vi "CANTESTDouble.vi"(6 "Data Input(Hex)":string="000007d100000000", 8 "错误输入（无错误）":errorcluster, 9 "ID(Hex 高位有效)":string="00000182", 10 "CANChannel":u32) -> (0 "错误输出":errorcluster, 3 "帧数据":string)   [LabVIEW 2013]
uses:
  InitConfig.ctl
  DevType.ctl
panel:
  out "Result":bool
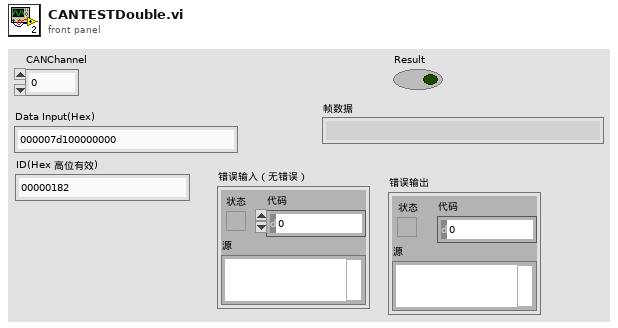
[diagram p1: front panel]
types:
  T1 = typedef "DevType.ctl" = u16
  T2 = typedef "InitConfig.ctl" = cluster{"AccCode":u32, "AccMask":u32, "Reserved":u32, "Filter":u8, "kCanBaud":u8, "Timing0":u8, "Timing1":u8, "Mode":u8, "CanRx_IER":u8}
  T3 = cluster{"ID":u8, u8, u8, u8, "TimeStamp":u32, "TimeFlag":u8, "SendType":u8, "RemoteFlag":u8, "ExternFlag":u8, "DataLen":u8, "Byte0":u8, "Byte1":u8, "Byte2":u8, "Byte3":u8, "Byte4":u8, "Byte5":u8, "Byte6":u8, "Byte7":u8, "Channel":u8, u8, u8}
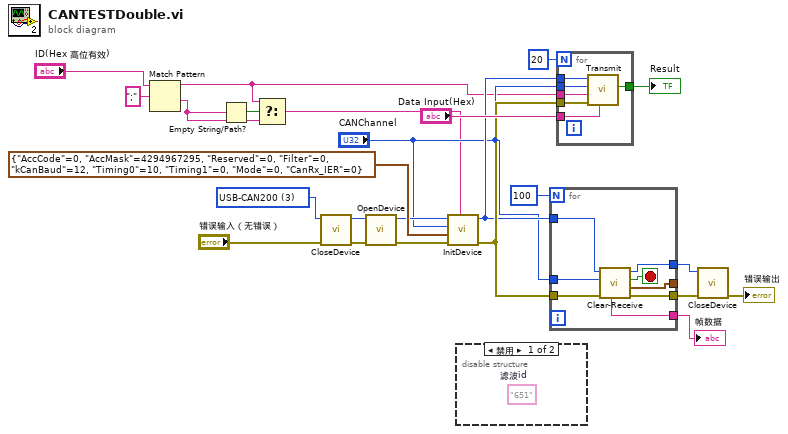
[diagram p0: block diagram]
diagram:
  w23 = T1 3 items=["PCI-CAN200"=7, "USB-CAN"=2, "USB-CAN200"=3] ("DeviceType")
  n1 = Match Pattern(string="ID(Hex 高位有效)", regular expression=";" ("正则表达式")) -> (before substring=w3:string, after substring=w2:string)  [unwired: 1 in, 2 out]
  n2 = Empty String/Path?(string/path=w2) -> (empty?=w4:bool)
  n3 = Select(t=w3, s=w4, f=w2) -> (s? t:f=w1:string)
  n4 = call "CloseDevice.vi"("错误输入（无错误）"="错误输入（无错误）", "DeviceType"=w23) -> ("错误输出"=w17:errorcluster, "DeviceTypeOut"=w22:u16)  [unwired: 7 in, 1 out]
  n5 = call "OpenDevice.vi"("错误输入（无错误）"=w17, "DeviceType"=w22) -> ("错误输出"=w18:errorcluster, "DeviceTypeOut"=w21:u16)  [unwired: 7 in, 1 out]
  n6 = call "InitDevice.vi"("ID(Hex 高位有效)"=w1, "错误输入（无错误）"=w18, "InitConfig"=T2 {"AccCode"=0, "AccMask"=4294967295, "Reserved"=0, "Filter"=0, "kCanBaud"=12, "Timing0"=10, "Timing1"=0, "Mode"=0, "CanRx_IER"=0}, "CanChannel"="CANChannel", "DeviceType"=w21) -> ("错误输出"=w12:errorcluster, "DeviceTypeOut"=w9:u16)  [unwired: 4 in, 1 out]
  n7 = disable-structure shown="禁用" {
    frame Disabled {
      (unwired) "651"  # 滤波id
    }
    frame Enabled {
    }
  }
  n8 = for {
    N: 100 -> [_]
    tunnel: "CANChannel" -> [w32]
    tunnel: w12 -> [w31]
    tunnel: [w29] -> _
    tunnel: [w28] -> w13
    tunnel: [w27] -> w11
    tunnel: w9 -> [w26]
    tunnel: [w25] -> w10
    stop <- w30 stop-if-true
    n9 = call "Clear-Receive.vi"("错误输入（无错误）"=w31, "CANChannel"=w32, "DeviceType"=w26) -> ("错误输出"=w28:errorcluster, "VCI_CAN_OBJ_R"=w29:T3, "Result"=w30:bool, "DeviceTypeOut"=w25:u16, "data"=w27:string)  [unwired: 2 in, 2 out]
  }
  "帧数据" <- w11
  n10 = for {
    N: 20 -> [_]
    tunnel: [w38] -> w20
    tunnel: w3 -> [w37]
    tunnel: "Data Input(Hex)" -> [w36]
    tunnel: "CANChannel" -> [w35]
    tunnel: w12 -> [w34]
    tunnel: w9 -> [w33]
    n11 = call "Transmit.vi"("Data Input(Hex)"=w36, "错误输入（无错误）"=w34, "ID(Hex 高位有效)"=w37, "CANChannel"=w35, "DeviceType"=w33) -> ("Result"=w38:bool)  [unwired: 4 in, 2 out]
  }
  "Result" <- w20
  n12 = call "CloseDevice.vi"("错误输入（无错误）"=w13, "DeviceType"=w10) -> ("错误输出"=→"错误输出":errorcluster)  [unwired: 7 in, 2 out]
